vi "LEDBreath.vi"() -> ()   [LabVIEW 2020]
uses:
  GlobalVariables.vi
panel:
  in  "Color":enum16{"Green", "Orange"}(ring)
  in  "Stop":bool
  out "Error Out":errorcluster
  in  "Error In":errorcluster
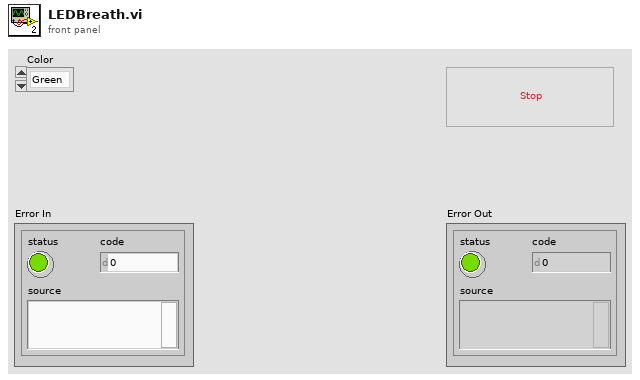
[diagram p1: front panel]
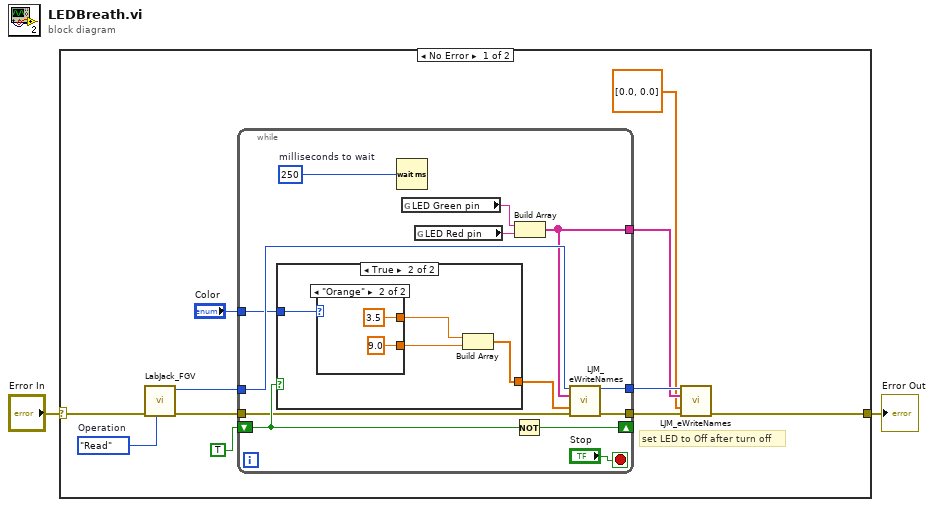
[diagram p0: block diagram]
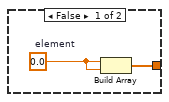
[diagram p2: hidden frame]
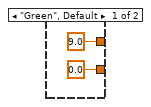
[diagram p3: hidden frame]
diagram:
  n1 = case shown="No Error" "Error In" {
    selector: "Error In" -> [w13 w37]
    tunnel: [w6 w37] -> w2
    frame No Error {
      w12 = enum16{"Write", "Read"}."Read"  # Operation
      # "set LED to Off after turn off"
      n2 = call "LabJack_FGV.vi"("Operation(Read)"=w12, "error in (no error)"=w13) -> ("error out"=w9:errorcluster, "Read data"=w11:i32)  [unwired: 8 in]
      n3 = while {
        tunnel: w11 -> [w24]
        shift-right: [w21] -> _
        shift-left: TRUE -> [w20]
        tunnel: w9 -> [w18]
        tunnel: [w17] -> w7
        tunnel: "Color" -> [w16]
        tunnel: [w15] -> w5
        tunnel: [w14] -> w4
        stop <- "Stop" stop-if-true
        w25 = u32 250  # milliseconds to wait
        n4 = case shown="True" w20 {
          tunnel: [w28 w31] -> w19
          tunnel: w16 -> [_ w29]
          frame False {
            w27 = 0.0  # element
            n5 = Build Array(w27, w27) -> (w28:dbl[])
          }
          frame True {
            n6 = case shown="\"Orange\"" w29 {
              tunnel: [9.0 ("element") 3.5 ("element")] -> w32
              tunnel: [0.0 ("element") 9.0 ("element")] -> w30
              frame "Green", Default {
              }
              frame "Orange" {
              }
            }
            n7 = Build Array(w32, w30) -> (w31:dbl[])
          }
        }
        n8 = Wait (ms)(milliseconds to wait=w25) -> ()  [unwired: 1 out]
        n9 = global read "GlobalVariables.vi" "LED Green pin"() -> (w23:string)
        n10 = global read "GlobalVariables.vi" "LED Red pin"() -> (w22:string)
        n11 = Not(x=w20) -> (.not. x?=w21:bool)
        n12 = Build Array(w23, w22) -> (w14:string[])
        n13 = call "LJM_eWriteNames.vi"("Handle In"=w24, "aNames"=w14, "aValuesIn"=w19, "error in"=w18) -> ("Handle Out"=w15:i32, "error out"=w17:errorcluster)  [unwired: 9 in, 1 out]
      }
      n14 = call "LJM_eWriteNames.vi"("Handle In"=w5, "aNames"=w4, "aValuesIn"=dbl[] [0.0, 0.0], "error in"=w7) -> ("error out"=w6:errorcluster)  [unwired: 9 in, 2 out]
    }
    frame Error {
    }
  }
  "Error Out" <- w2
